vi "Disable UI.vi"(8 "error in (no error)":errorcluster, 11 "Operator UI Actor in":refnum<class "Controller UI.lvclass">) -> (0 "error out":errorcluster, 3 "Operator UI Actor out":refnum<class "Controller UI.lvclass">)   [LabVIEW 2016, in "Controller UI.lvlib" / "Controller UI.lvclass"]
uses:
  <userlib>/Common Components/Controller UI/Controller UI.lvclass
  <userlib>/Common Components/Controller UI/Controller UI.lvclass/Controller UI.ctl
  <userlib>/Common Components/Controller UI/Accessors/Read View Results.vi
  <userlib>/Common Components/Controller UI/Accessors/Read Load New Function.vi
  <userlib>/Common Components/Controller UI/Accessors/Read Run.vi
  <userlib>/Common Components/Controller UI/Accessors/Read Function.vi
  <userlib>/Common Components/Controller UI/Accessors/Read Show FP_.vi
  <userlib>/Common Components/Controller UI/Accessors/Read Results Listbox.vi
  <userlib>/Common Components/User Interface/UI.lvclass
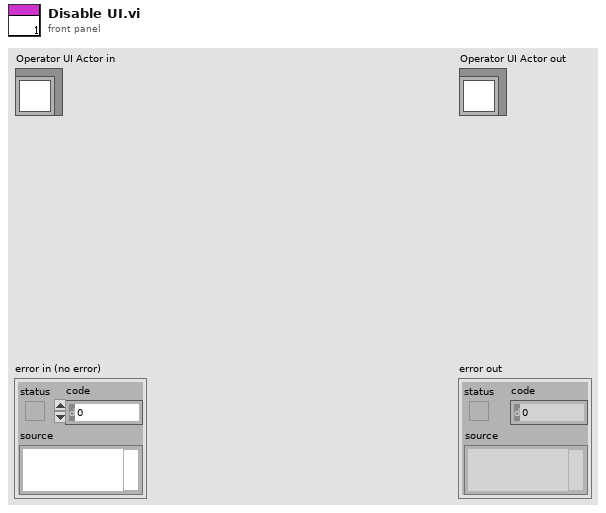
[diagram p1: front panel]
types:
  T1 = enum8{"Enabled", "Disabled", "Disabled and Grayed Out"}
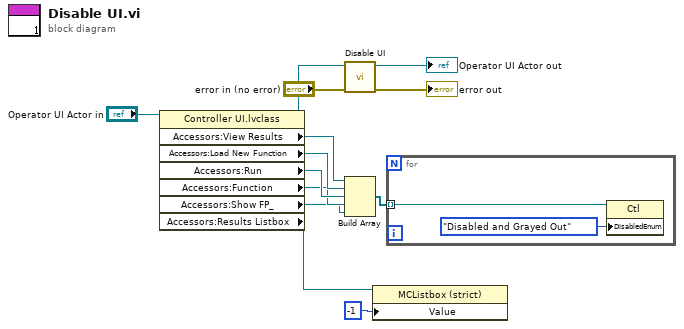
[diagram p0: block diagram]
diagram:
  n1 = property class="Controller UI.lvclass"(reference="Operator UI Actor in") -> (reference out=w8:refnum<class "Controller UI.lvclass">, "Accessors:View Results"=w7:refnum<vi>, "Accessors:Load New Function"=w6:refnum<vi>, "Accessors:Run"=w5:refnum<vi>, "Accessors:Function"=w4:refnum<vi>, "Accessors:Show FP_"=w3:refnum<vi>, "Accessors:Results Listbox"=w1:refnum<vi>)  [unwired: 1 in, 1 out]
  n2 = call-parent "Disable UI.vi"("error in (no error)"="error in (no error)", "UI in"=w8) -> ("error out"=→"error out":errorcluster, "UI out"=→"Operator UI Actor out":refnum<class "Controller UI.lvclass">)  [unwired: 8 in]
  n3 = Build Array(w7, w6, w5, w4, w3) -> (w10:refnum<vi>[])
  n4 = property class="MCListbox (strict)"(reference=w1, "Value"=-1 ("Listbox")) -> ()  [unwired: 1 in, 2 out]
  n5 = for {
    tunnel: w10 -> [w15] mode=indexing
    n6 = property class="Ctl"(reference=w15, "DisabledEnum"=T1."Disabled and Grayed Out" ("Disabled")) -> ()  [unwired: 1 in, 2 out]
  }
